vi "Extend pulse width.vi"(7 "Function":enum16{"Minimum width", "Exact width"}(ring)=enum."Exact width", 9 "Pulse width (ticks)(80000=1ms @80MHz)":u32=80000, 11 "Input signal":bool) -> (3 "Output signal":bool)   [LabVIEW 2020]
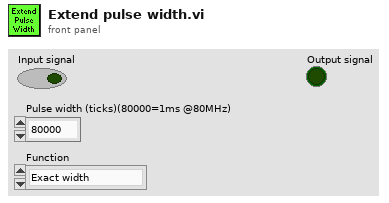
[diagram p1: front panel]
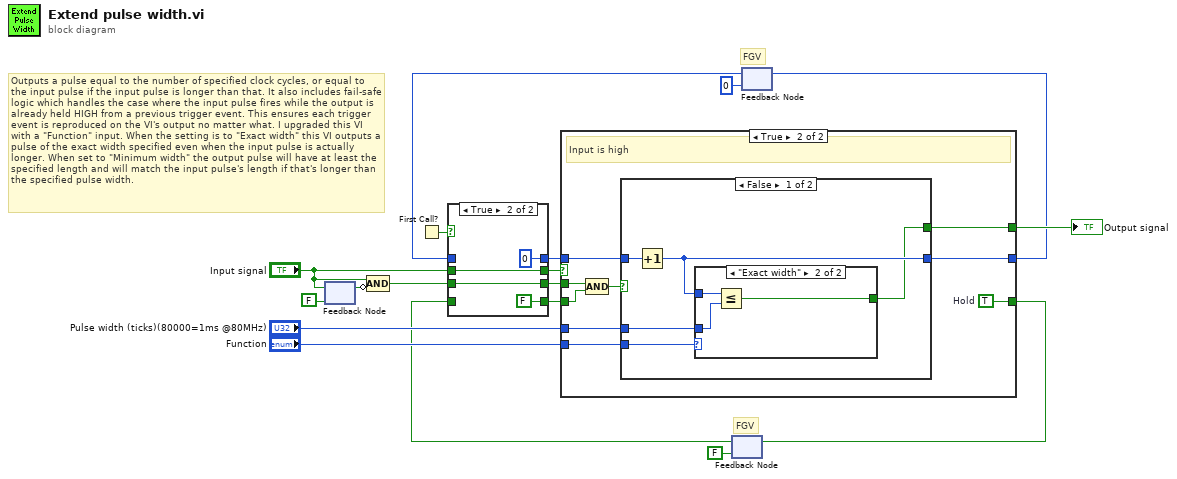
[diagram p0: block diagram]
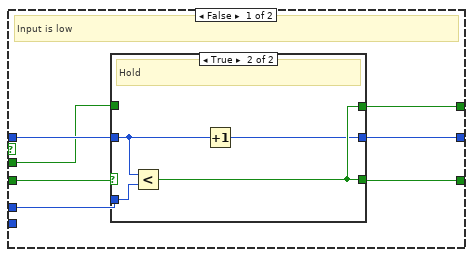
[diagram p3: hidden frame]
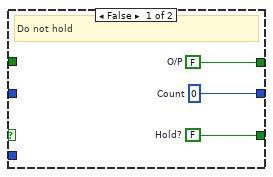
[diagram p4: hidden frame]
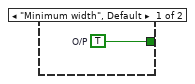
[diagram p5: hidden frame]
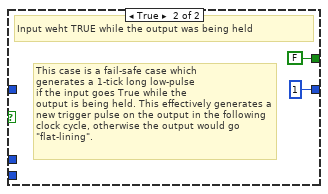
[diagram p6: hidden frame]
diagram:
  # "FGV"
  # "FGV"
  # "Outputs a pulse equal to the number of specified clock cycles, or equal to the input pulse if the input pulse is longer than that. It also includes fail-safe logic which handles the case where the input pulse fires while the output is already held HIGH from a previous trigger event. This ensures each trigger event is reproduced on the VI's output no matter what. I upgraded this VI with a \"Function\" input. When the setting is to \"Exact width\" this VI outputs a pulse of the exact width specified even when the input pulse is actually longer. When set to \"Minimum width\" the output pulse will have at least the specified length and will match the input pulse's length if that's longer than the specified pulse width."
  n1 = feedback-in #1("Input signal") -> ()
  n2 = feedback #1(FALSE ("Hold")) -> (w16:bool)
  n3 = Compound Arithmetic op=AND("Input signal", invert w16) -> (w15:bool)
  n4 = First Call?() -> (First Call?: T/F=w5:bool)
  n5 = feedback #2(FALSE ("Hold")) -> (w8:bool)
  n6 = feedback #3(u32 0 ("Count")) -> (w10:u32)
  n7 = case shown="True" w5 {
    tunnel: w10 -> [w22 _]
    tunnel: [w22 u32 0 ("Count")] -> w4
    tunnel: w8 -> [w21 _]
    tunnel: [w21 FALSE ("Hold")] -> w3
    tunnel: [w20 w25] -> w2
    tunnel: w15 -> [w20 w25]
    tunnel: [w19 w26] -> w1
    tunnel: "Input signal" -> [w19 w26]
    frame False {
    }
    frame True {
    }
  }
  n8 = case shown="True" w1 {
    tunnel: [w28 w48] -> w11
    tunnel: w4 -> [w32 w49]
    tunnel: [w31 w43] -> w18
    tunnel: "Pulse width (ticks)(80000=1ms @80MHz)" -> [w33 w42]
    tunnel: [w29 w47] -> w9
    tunnel: w3 -> [w30 w45]
    tunnel: w2 -> [w27 w46]
    tunnel: "Function" -> [_ w41]
    frame False {
      # "Input is low"
      n9 = case shown="True" w30 {
        tunnel: w33 -> [_ w40]
        tunnel: w32 -> [_ w38]
        tunnel: [w35 w39] -> w31
        tunnel: [w36 w39] -> w29
        tunnel: [w34 w37] -> w28
        tunnel: w27 -> [_ _]
        frame False {
          w34 = u32 0  # Count
          w35 = FALSE  # O/P
          w36 = FALSE  # Hold?
          # "Do not hold"
        }
        frame True {
          # "Hold"
          n10 = Less?(x=w38, y=w40) -> (x < y?=w39:bool)
          n11 = Increment(x=w38) -> (x+1=w37:u32)
        }
      }
    }
    frame True {
      w47 = TRUE  # Hold
      # "Input is high"
      n12 = Compound Arithmetic op=AND(w46, w45) -> (w44:bool)
      n13 = case shown="False" w44 {
        tunnel: w49 -> [w54 _]
        tunnel: [w53 u32 1] -> w48
        tunnel: [w51 FALSE ("O/P")] -> w43
        tunnel: w42 -> [w52 _]
        tunnel: w41 -> [w50 _]
        frame False {
          n14 = Increment(x=w54) -> (x+1=w53:u32)
          n15 = case shown="\"Exact width\"" w50 {
            tunnel: w53 -> [_ w58]
            tunnel: w52 -> [_ w57]
            tunnel: [w55 w56] -> w51
            frame "Minimum width", Default {
              w55 = TRUE  # O/P
            }
            frame "Exact width" {
              n16 = Less Or Equal?(x=w58, y=w57) -> (x <= y?=w56:bool)
            }
          }
        }
        frame True {
          # "This case is a fail-safe case which\ngenerates a 1-tick long low-pulse\nif the input goes True while the\noutput is being held. This effectively generates a new trigger pulse on the output in the following clock cycle, otherwise the output would go \"flat-lining\"."
          # "Input weht TRUE while the output was being held"
        }
      }
    }
  }
  "Output signal" <- w18
  n17 = feedback-in #2(w9) -> ()
  n18 = feedback-in #3(w11) -> ()
